vi "3SistemasCal.vi"() -> ()   [LabVIEW 2010]
uses:
  <vilib>/vision/NI_Vision_Development_Module.lvlib
  <vilib>/vision/driver/NI_Vision_Acquisition_Software.lvlib
  Program Files/National Instruments/LabVIEW 2010/resource/objmgr/imaqdx.rc
panel:
  out "Template":T1(plugin-control)
  out "Image":T1(plugin-control)
  out "Tamanho da linha":dbl
  out "Ajuste de centimetos\npor pixels":dbl
  in  "Distãncia de ajuste\nem centrimetos":dbl=25.0
  in  "Palette:Palette Type":u32(ring) items=["Grayscale", "Binary", "Gradient", "Rainbow", "Temperature", "User Defined"]
  out "error out":errorcluster
  in  "Zoom to Fit\nTemplate":bool=TRUE
  out "AcquisitionInProgress":bool
  in  "VideoMode":u32
  out "Meter":dbl(knob) scale=0.0..100.0 scale format="%.1f"
  out "processed FPS":dbl
  in  "Camera escolhida":i32
  out "Nome \nCamera":T2
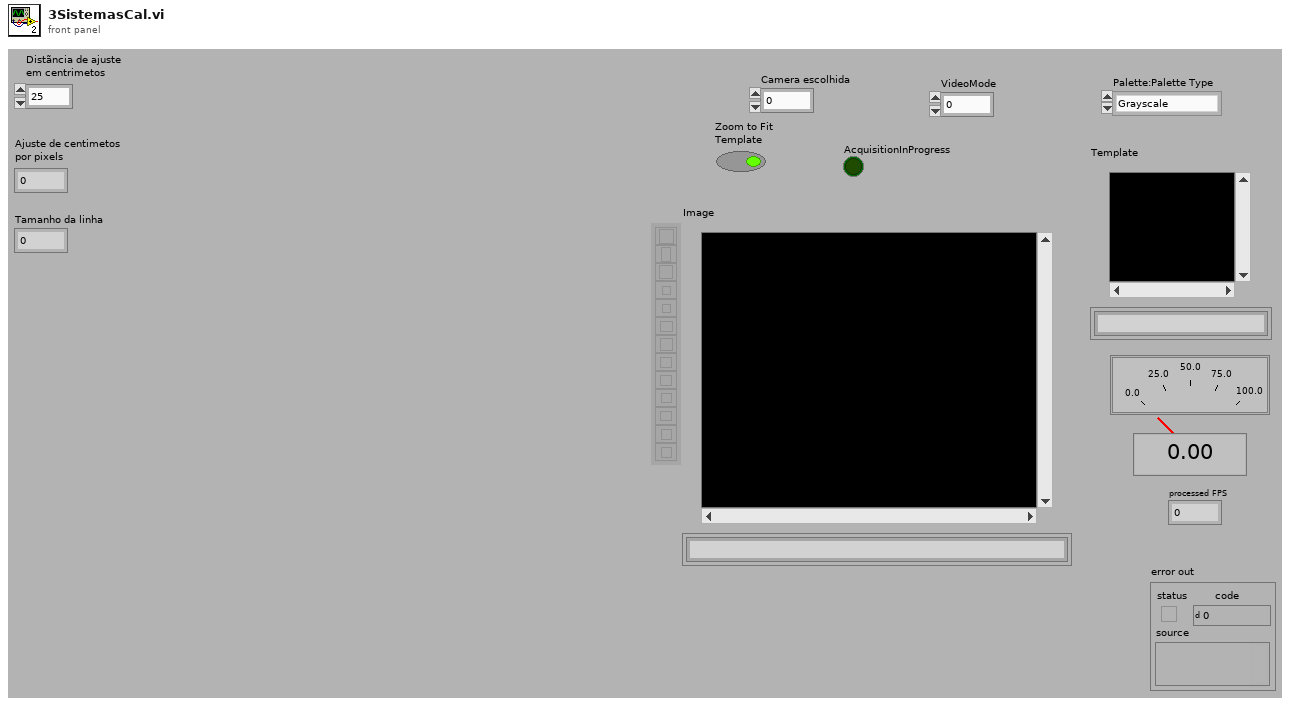
[diagram p1: front panel]
types:
  T1 = typedef "IMAQ Image.ctl" = refnum<image>
  T2 = cluster{"Type":u32, "Version":u32, "Flags":u32, "SerialNumberHigh":u32, "SerialNumberLow":u32, "BusType":u32, "InterfaceName":string, "VendorName":string, "ModelName":string, "CameraFileName":string, "CameraAttributeURL":string}
  T3 = typedef "Image Type" = u32
  T4 = cluster{"Type":u32, "Version":u32, "Flags":u32, "SerialNumberHigh":u32, "SerialNumberLow":u32, "BusType":u32, "InterfaceName":string, "VendorName":string, "ModelName":string, "CameraFileName":string, "CameraAttributeURL":string}[]
  T5 = typedef "IMAQdx.ctl" = refnum<k21>
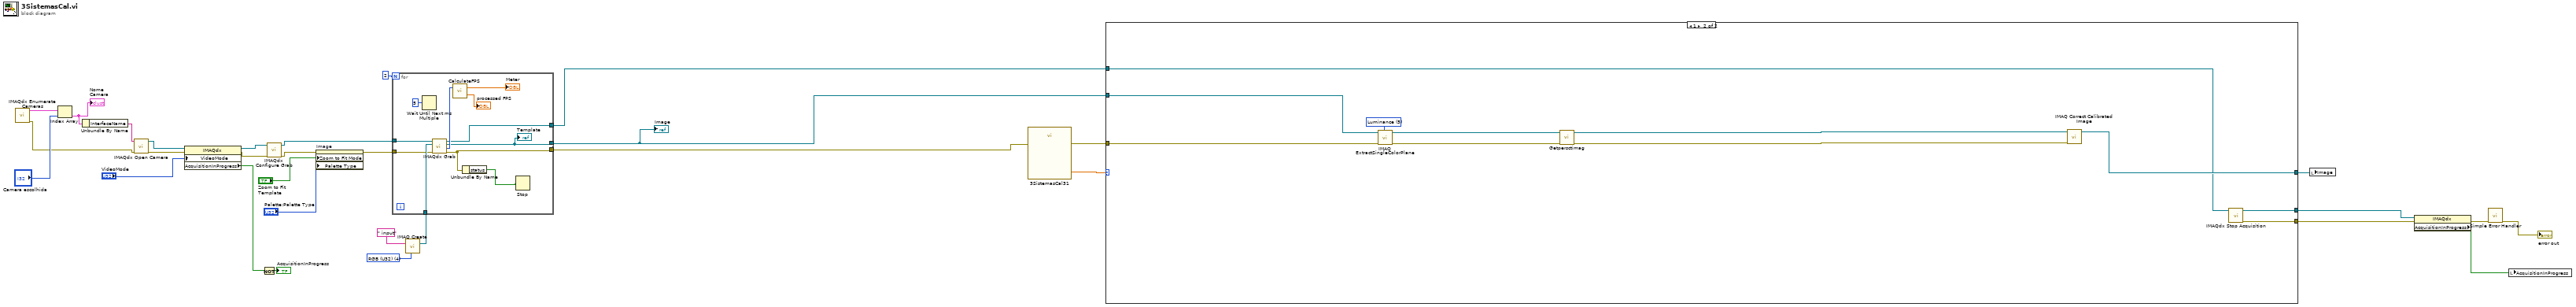
[diagram p0: block diagram]
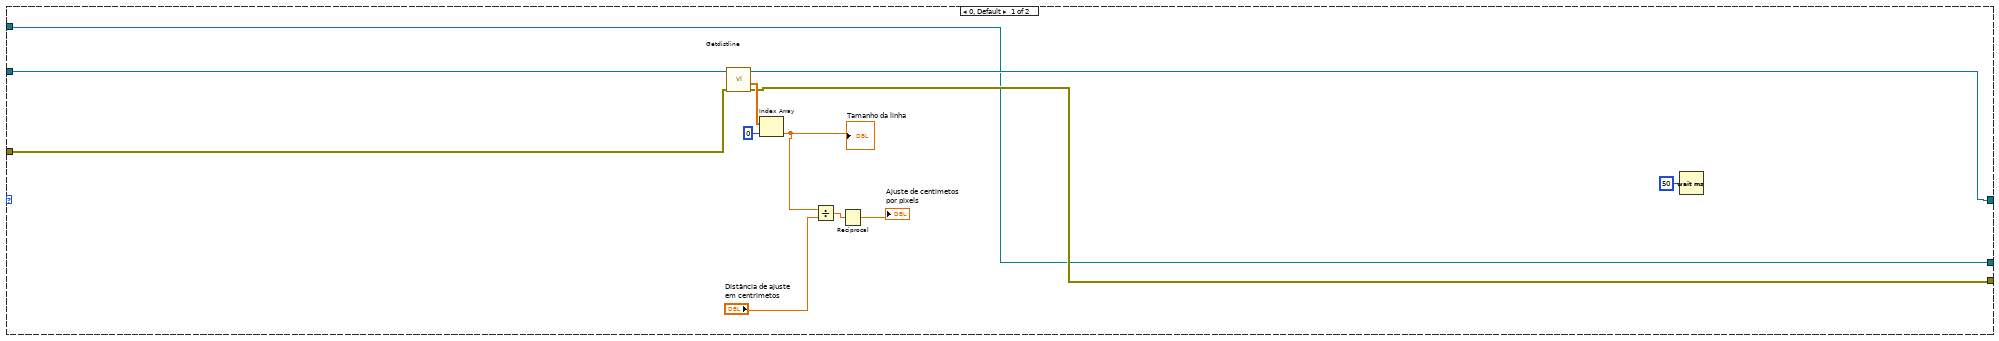
[diagram p2: hidden frame]
diagram:
  w27 = T3 4 items=["Grayscale (U8)", "Grayscale (I16)", "Grayscale (SGL)", "Complex (CSG)", "RGB (U32)", "HSL (U32)", "RGB (U64)"] ("Image Type")
  n1 = call <vilib>:"IMAQdx Enumerate Cameras.vi"() -> ("error out"=w25:errorcluster, "Camera Information Array"=w31:T4)  [unwired: 10 in]
  n2 = Index Array(array=w31, index="Camera escolhida") -> (element=w24:T2)
  "Nome \nCamera" <- w24
  n3 = Unbundle By Name(w24) -> ("InterfaceName"=w23:string)
  n4 = call <vilib>:"IMAQdx Open Camera.vi"("error in"=w25, "Session In"=w23) -> ("error out"=w29:errorcluster, "Session Out"=w22:T5)  [unwired: 8 in]
  n5 = property class="IMAQdx"(reference=w22, error in=w29, "VideoMode"="VideoMode") -> (reference out=w17:T5, error out=w15:errorcluster, "AcquisitionInProgress"=w20:bool)
  n6 = Not(x=w20) -> (.not. x?=→"AcquisitionInProgress":bool)
  n7 = call <vilib>:"IMAQdx Configure Grab.vi"("error in"=w15, "Session In"=w17) -> ("error out"=w6:errorcluster, "Session Out"=w16:T5)  [unwired: 8 in]
  n8 = property on="Image" class="ImageControl"(error in=w6, "Zoom to Fit Mode"="Zoom to Fit\nTemplate", "Palette Type"="Palette:Palette Type") -> (error out=w5:errorcluster)  [unwired: 1 in, 1 out]
  n9 = call "IMAQ Create"("Image Name"=" input", "Image Type"=w27) -> ("New Image"=w26:T1)  [unwired: 3 in, 1 out]
  n10 = for {
    N: 2 -> [_]
    tunnel: w26 -> [w43]
    tunnel: w16 -> [w42]
    tunnel: w5 -> [w41]
    tunnel: [w40] -> w13
    tunnel: [w33] -> w9
    tunnel: [w34] -> w10
    n11 = Wait Until Next ms Multiple(millisecond multiple=u32 5 ("milliseconds to wait")) -> ()  [unwired: 1 out]
    n12 = call <vilib>:"IMAQdx Grab.vi"("error in"=w41, "Image In"=w43, "Session In"=w42) -> ("error out"=w40:errorcluster, "Buffer Number Out"=w39:u32, "Image Out"=w33:T1, "Session Out"=w34:T5)  [unwired: 5 in]
    "Template" <- w33
    n13 = call "CalculateFPS.vi"("buffer number"=w39) -> ("processed FPS"=→"processed FPS":dbl, "acquired FPS"=→"Meter":dbl)  [unwired: 1 in]
    n14 = Unbundle By Name(w40) -> ("status"=w35:bool)
    n15 = Stop(stop? (T)=w35) -> ()
  }
  "Image" <- w9
  n16 = call "3SistemasCal31.vi"("error in (no error)"=w13) -> ("Tipo de Calibração"=w32:dbl, "error out"=w14:errorcluster)  [unwired: 16 in, 1 out]
  n17 = case shown="1" w32 {
    tunnel: w9 -> [w48 w65]
    tunnel: w14 -> [w47 w64]
    tunnel: [w46 w63] -> w2
    tunnel: w10 -> [w44 w60]
    tunnel: [w45 w61] -> w8
    tunnel: [w44 w62] -> w1
    frame 0, Default {
      n18 = call "Getdistline.vi"("error in"=w47, "Image in"=w48) -> ("error out"=w46:errorcluster, "Comprimento\nem pixels"=w53:dbl[], "Image out"=w45:T1)  [unwired: 6 in]
      n19 = Index Array(array=w53, index=0) -> (element=w50:dbl)
      "Tamanho da linha" <- w50
      n20 = Divide(x=w50, y="Distãncia de ajuste\nem centrimetos") -> (x/y=w51:dbl)
      n21 = Reciprocal(x=w51) -> (1/x=→"Ajuste de centimetos\npor pixels":dbl)
      n22 = Wait (ms)(milliseconds to wait=u32 50) -> ()  [unwired: 1 out]
    }
    frame 1 {
      w66 = 5 items=["Red", "Green", "Blue", "Hue", "Saturation", "Luminance", "Value", "Intensity"] ("Color Plane")
      n23 = call "IMAQ ExtractSingleColorPlane"("Color Plane"=w66, "error in (no error)"=w64, "Image Src"=w65) -> ("error out"=w58:errorcluster, "Image Dst Out"=w59:T1)  [unwired: 1 in, 6 out]
      n24 = call "Getpersctimag.vi"("error in"=w58, "Image in"=w59) -> ("error out"=w56:errorcluster, "Image out"=w57:T1)  [unwired: 8 in]
      n25 = call "IMAQ Correct Calibrated Image"("error in (no error)"=w56, "Image Src"=w57) -> ("Corrected Image"=w61:T1)  [unwired: 8 in, 1 out]
      n26 = call <vilib>:"IMAQdx Stop Acquisition.vi"("Session In"=w60) -> ("error out"=w63:errorcluster, "Session Out"=w62:T5)  [unwired: 9 in]
    }
  }
  n27 = local write "Image"(w8) -> ()
  n28 = property class="IMAQdx"(reference=w1, error in=w2) -> (error out=w12:errorcluster, "AcquisitionInProgress"=w7:bool)  [unwired: 1 out]
  n29 = call <vilib>:"Simple Error Handler.vi"("error in (no error)"=w12) -> ("error out"=→"error out":errorcluster)  [unwired: 4 in, 4 out]
  n30 = local write "AcquisitionInProgress"(w7) -> ()
